vi "test_find_elements.vi"() -> ()   [LabVIEW 2016]
uses:
  find_element(array).vi
  find_element(variant).vi
panel:
  out "elapsed time in millisec (variant)":dbl
  out "elapsed time in millisec (array)":dbl
  in  "number of elements":i32=10000
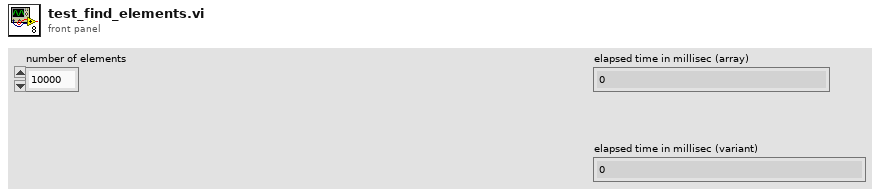
[diagram p1: front panel]
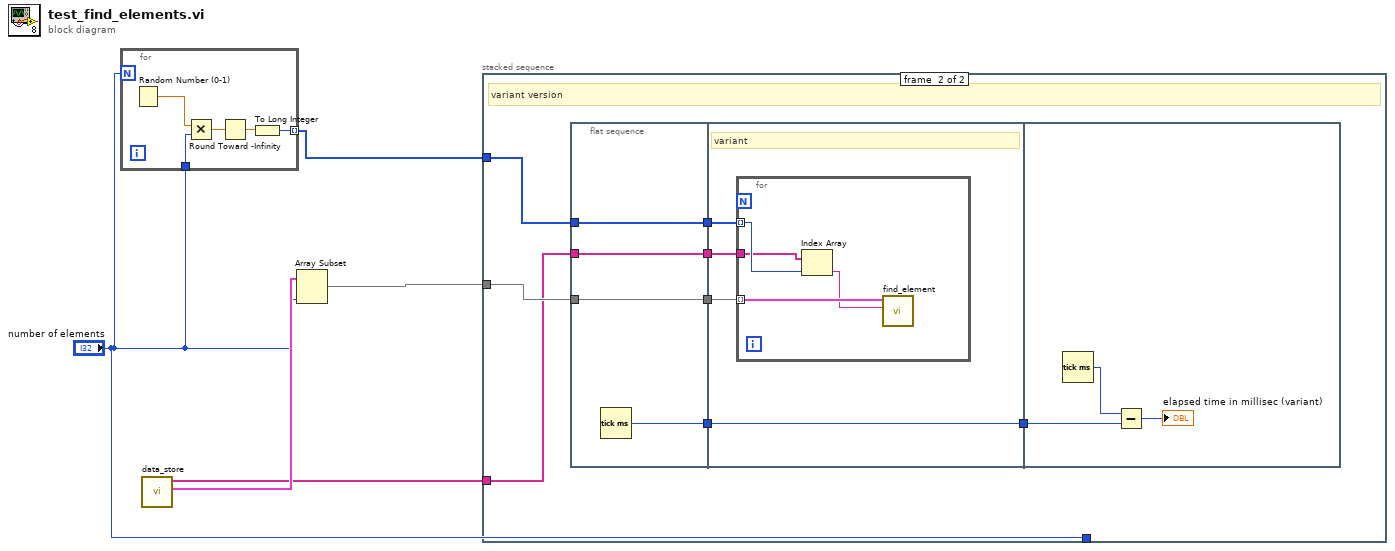
[diagram p0: block diagram]
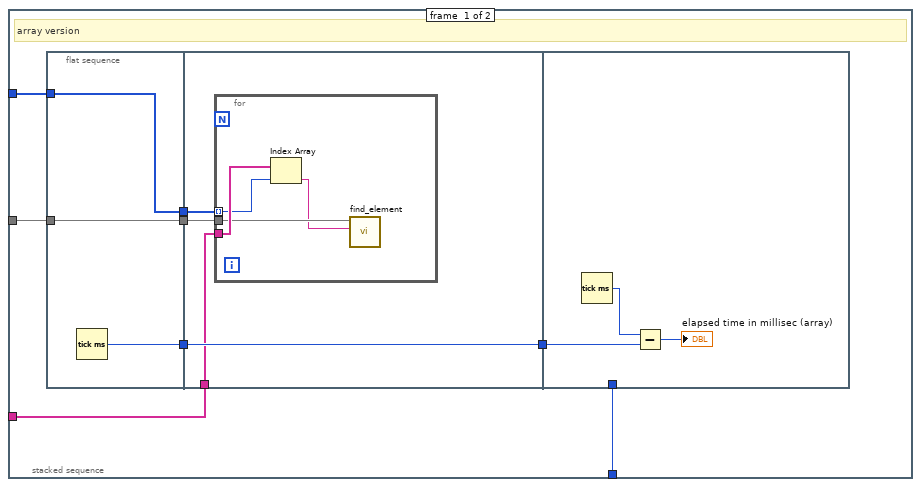
[diagram p2: hidden frame]
diagram:
  n1 = for {
    N: "number of elements" -> [_]
    tunnel: "number of elements" -> [w10]
    tunnel: [w6] -> w1 mode=indexing
    n2 = Random Number (0-1)() -> (number: 0 to 1=w9:dbl)
    n3 = Multiply(x=w9, y=w10) -> (x*y=w8:dbl)
    n4 = Round Toward -Infinity(1:w8) -> (0:w7:dbl)
    n5 = To Long Integer(number=w7) -> (32bit integer=w6:i32)
  }
  n6 = call "data_store.vi"() -> ("array items"=w5:cluster{"name":string, "address":string}[], "names"=w2:string[])  [unwired: 10 in]
  n7 = Array Subset(array=w5, length="number of elements") -> (w4:cluster{"name":string, "address":string}[])  [unwired: 1 in]
  n8 = stacked-sequence {
    tunnel: "number of elements" -> [w15 _]
    tunnel: w4 -> [w14 w37]
    tunnel: w2 -> [w13 w34]
    tunnel: w1 -> [w12 w36]
    frame #0 {
      # "array version"
      n9 = flat-sequence {
        tunnel: [w21] -> w18
        tunnel: w14 -> [w20]
        tunnel: [w20] -> w17
        tunnel: w12 -> [w19]
        tunnel: [w19] -> w11
        tunnel: [w25] -> w16
        tunnel: w18 -> [w25]
        tunnel: w17 -> [w24]
        tunnel: w13 -> [w23]
        tunnel: w11 -> [w22]
        tunnel: w16 -> [w31]
        tunnel: w15 -> [_]
        frame #0 {
          n10 = Tick Count (ms)() -> (millisecond timer value=w21:u32)
        }
        frame #1 {
          n11 = for {
            tunnel: w24 -> [w27]
            tunnel: w23 -> [w29]
            tunnel: w22 -> [w28] mode=indexing
            n12 = Index Array(array=w29, index=w28) -> (element=w26:string)
            n13 = call-poly "find_element.vi"("name"=w26, "data store (in)"=w27) -> ()  [unwired: 6 in, 4 out]
          }
        }
        frame #2 {
          n14 = Tick Count (ms)() -> (millisecond timer value=w32:u32)
          n15 = Subtract(x=w32, y=w31) -> (x-y=→"elapsed time in millisec (array)":u32)
        }
      }
    }
    frame #1 {
      # "variant version"
      n16 = flat-sequence {
        tunnel: [w44] -> w40
        tunnel: w37 -> [w43]
        tunnel: [w43] -> w39
        tunnel: w36 -> [w42]
        tunnel: [w42] -> w35
        tunnel: w34 -> [w41]
        tunnel: [w41] -> w33
        tunnel: [w48] -> w38
        tunnel: w40 -> [w48]
        tunnel: w39 -> [w47]
        tunnel: w35 -> [w46]
        tunnel: w33 -> [w45]
        tunnel: w38 -> [w54]
        frame #0 {
          n17 = Tick Count (ms)() -> (millisecond timer value=w44:u32)
        }
        frame #1 {
          # "variant"
          n18 = for {
            tunnel: w47 -> [w52] mode=indexing
            tunnel: w46 -> [w51] mode=indexing
            tunnel: w45 -> [w50]
            n19 = Index Array(array=w50, index=w51) -> (element=w49:string)
            n20 = call-poly "find_element.vi"("name"=w49, "data store (in)"=w52) -> ()  [unwired: 6 in, 4 out]
          }
        }
        frame #2 {
          n21 = Tick Count (ms)() -> (millisecond timer value=w55:u32)
          n22 = Subtract(x=w55, y=w54) -> (x-y=→"elapsed time in millisec (variant)":u32)
        }
      }
    }
  }
